vi "GetDeviceIdentification.vi"(8 "error in":errorcluster, 11 "VISA resource name":refnum<visa-resource-name>) -> (0 "error out":errorcluster, 2 "8800 Response Identification":string, 3 "VISA resource name out":refnum<visa-resource-name>)   [LabVIEW 2023, in "Thermotron 8800.lvlib"]
doc: "IDEN\nCommand name: Send device identification\nCommand type: System status\nDescription: The 8800 sends an ASCII character string to the host computer.\nSyntax: IDEN?\nData type: ASCII character string\nQuery example: IDEN?\n8800 response: 8800 CHAMBER CONTROLLER"
uses:
  Thermotron 8800.lvlib
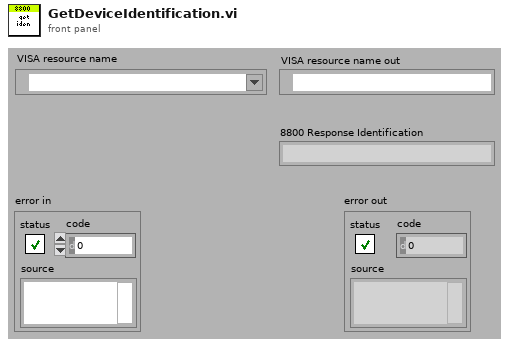
[diagram p1: front panel]
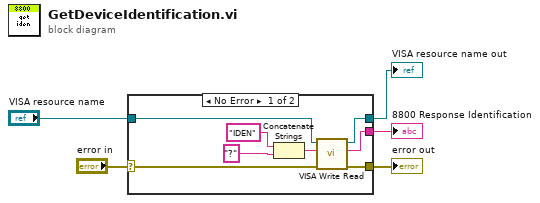
[diagram p0: block diagram]
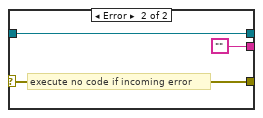
[diagram p2: hidden frame]
diagram:
  n1 = case shown="No Error" "error in" {
    selector: "error in" -> [w11 w16]
    tunnel: [w9 w16] -> w1
    tunnel: [w10 w15] -> w2
    tunnel: "VISA resource name" -> [w12 w15]
    tunnel: [w8 ""] -> w5
    frame No Error {
      n2 = Concatenate Strings("IDEN" ("8800 Command"), "?" ("8800 Command")) -> (w13:string)
      n3 = call "VISA Write Read.vi"("error in (no error)"=w11, "8800 Command"=w13, "VISA Refnum in"=w12) -> ("error out"=w9:errorcluster, "read buffer"=w8:string, "VISA Refnum out"=w10:refnum<visa-resource-name>)  [unwired: 6 in]
    }
    frame Error {
      # "execute no code if incoming error"
    }
  }
  "VISA resource name out" <- w2
  "error out" <- w1
  "8800 Response Identification" <- w5
